vi "CalculateSweepRate_xyz.vi"(8 "error in (no error)":errorcluster, 9 "Sweep rate (T/min)":dbl, 10 "B target":T3, 11 "B initial":T2) -> (0 "error out":errorcluster, 1 "time (min)":dbl, 3 "Sweep Rates":T1)   [LabVIEW 2016]
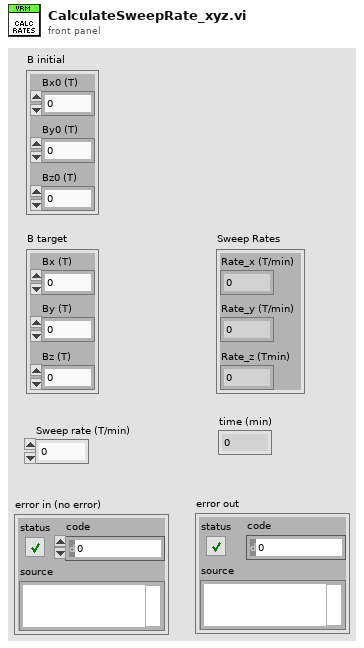
[diagram p1: front panel]
types:
  T1 = cluster{"Rate_x (T/min)":dbl, "Rate_y (T/min)":dbl, "Rate_z (Tmin)":dbl}
  T2 = cluster{"Bx0 (T)":dbl, "By0 (T)":dbl, "Bz0 (T)":dbl}
  T3 = cluster{"Bx (T)":dbl, "By (T)":dbl, "Bz (T)":dbl}
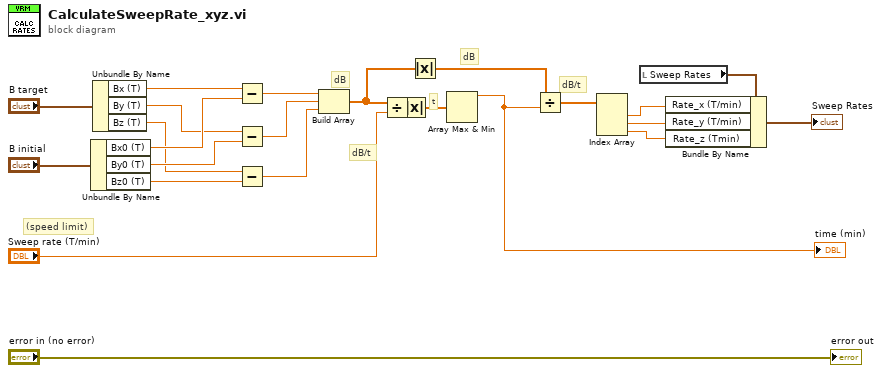
[diagram p0: block diagram]
diagram:
  # "dB/t"
  # "dB"
  # "(speed limit)"
  # "t"
  # "dB/t"
  # "dB"
  n1 = Unbundle By Name("B initial") -> ("Bx0 (T)"=w21:dbl, "By0 (T)"=w19:dbl, "Bz0 (T)"=w17:dbl)
  n2 = Unbundle By Name("B target") -> ("Bx (T)"=w22:dbl, "By (T)"=w20:dbl, "Bz (T)"=w18:dbl)
  n3 = Subtract(x=w22, y=w21) -> (x-y=w12:dbl)
  n4 = Subtract(x=w20, y=w19) -> (x-y=w14:dbl)
  n5 = Subtract(x=w18, y=w17) -> (x-y=w13:dbl)
  n6 = Build Array(w12, w14, w13) -> (w9:dbl[])
  n7 = Divide(x=w9, y="Sweep rate (T/min)") -> (x/y=w15:dbl[])
  n8 = Absolute Value(x=w15) -> (abs(x)=w2:dbl[])
  n9 = Absolute Value(x=w9) -> (abs(x)=w1:dbl[])
  n10 = Array Max & Min(array=w2) -> (max value=w11:dbl)  [unwired: 3 out]
  "time (min)" <- w11
  n11 = Divide(x=w1, y=w11) -> (x/y=w10:dbl[])
  n12 = Index Array(array=w10) -> (element #1=w8:dbl, element #2=w7:dbl, element #3=w6:dbl)  [unwired: 3 in]
  n13 = local read "Sweep Rates"() -> (w5:T1)
  n14 = Bundle By Name(cluster=w5, "Rate_x (T/min)"=w8, "Rate_y (T/min)"=w7, "Rate_z (Tmin)"=w6) -> (→"Sweep Rates":T1)
  "error out" <- "error in (no error)"
